vi "JJMCclase10.vi"() -> ()   [LabVIEW 2013]
panel:
  in  "detener programa":bool
  in  "llave":bool
  in  "llenar":bool
  out "tanque":i32(slide) scale=0.0..1000.0
  # "EVENTOS"
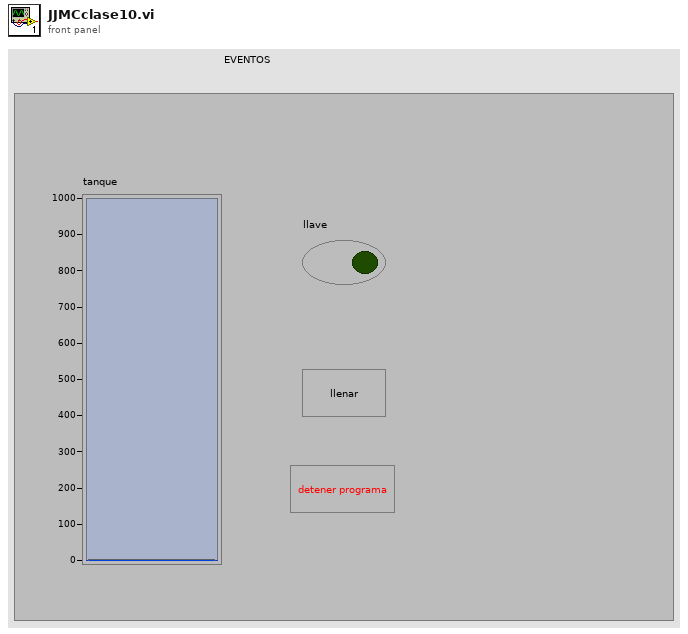
[diagram p1: front panel]
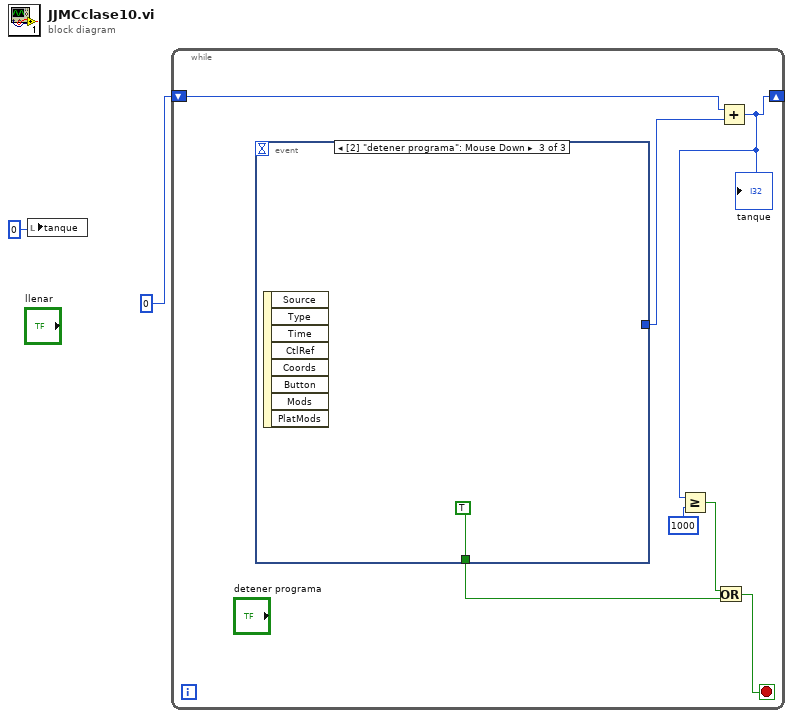
[diagram p0: block diagram]
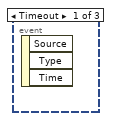
[diagram p2: hidden frame]
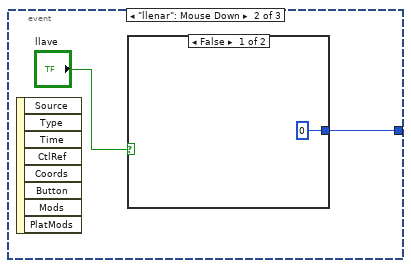
[diagram p3: hidden frame]
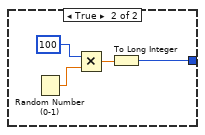
[diagram p4: hidden frame]
diagram:
  n1 = local write "tanque"(0) -> ()
  n2 = while {
    shift-right: [w7] -> _
    shift-left: 0 -> [w9]
    stop <- w4 stop-if-true
    n3 = event shown="[2] \"detener programa\": Mouse Down" {
      selector: _ -> [_ _ _]
      dyn-events: _ -> [_ _ _]
      timeout: _ -> [_ _ _]
      tunnel: [_ w10 _] -> w8
      tunnel: [_ _ TRUE] -> w3
      event Timeout {
        n4 = event-data() -> ()  [unwired: 1 in, 3 out]
      }
      event "llenar": Mouse Down {
        n5 = event-data() -> ()  [unwired: 1 in, 8 out]
        n6 = case shown="False" "llave" {
          tunnel: [0 w13] -> w10
          frame False {
          }
          frame True {
            n7 = Random Number (0-1)() -> (number: 0 to 1=w15:dbl)
            n8 = Multiply(x=100, y=w15) -> (x*y=w14:dbl)
            n9 = To Long Integer(number=w14) -> (32bit integer=w13:i32)
          }
        }
      }
      event "detener programa": Mouse Down {
        n10 = event-data() -> ()  [unwired: 1 in, 8 out]
      }
    }
    n11 = Add(x=w9, y=w8) -> (x+y=w7:i32)
    "tanque" <- w7
    n12 = Greater Or Equal?(x=w7, y=1000) -> (x >= y?=w5:bool)
    n13 = Or(x=w5, y=w3) -> (x .or. y?=w4:bool)
  }
